vi "Format Serial Data.vi"(0 "Time Stamp":timestamp, 5 "Bus Time":timestamp, 7 "Rail":i32, 9 "String":string, 11 "Error IN":errorcluster, 12 "#of Element Read":i32) -> (4 "Formatted Data":string[](array[string]), 15 "Error OUT":errorcluster)   [LabVIEW 2011]
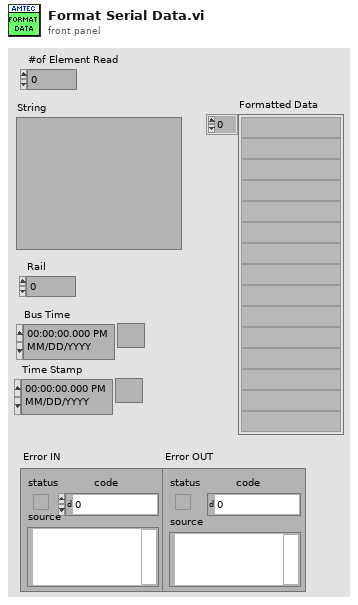
[diagram p1: front panel]
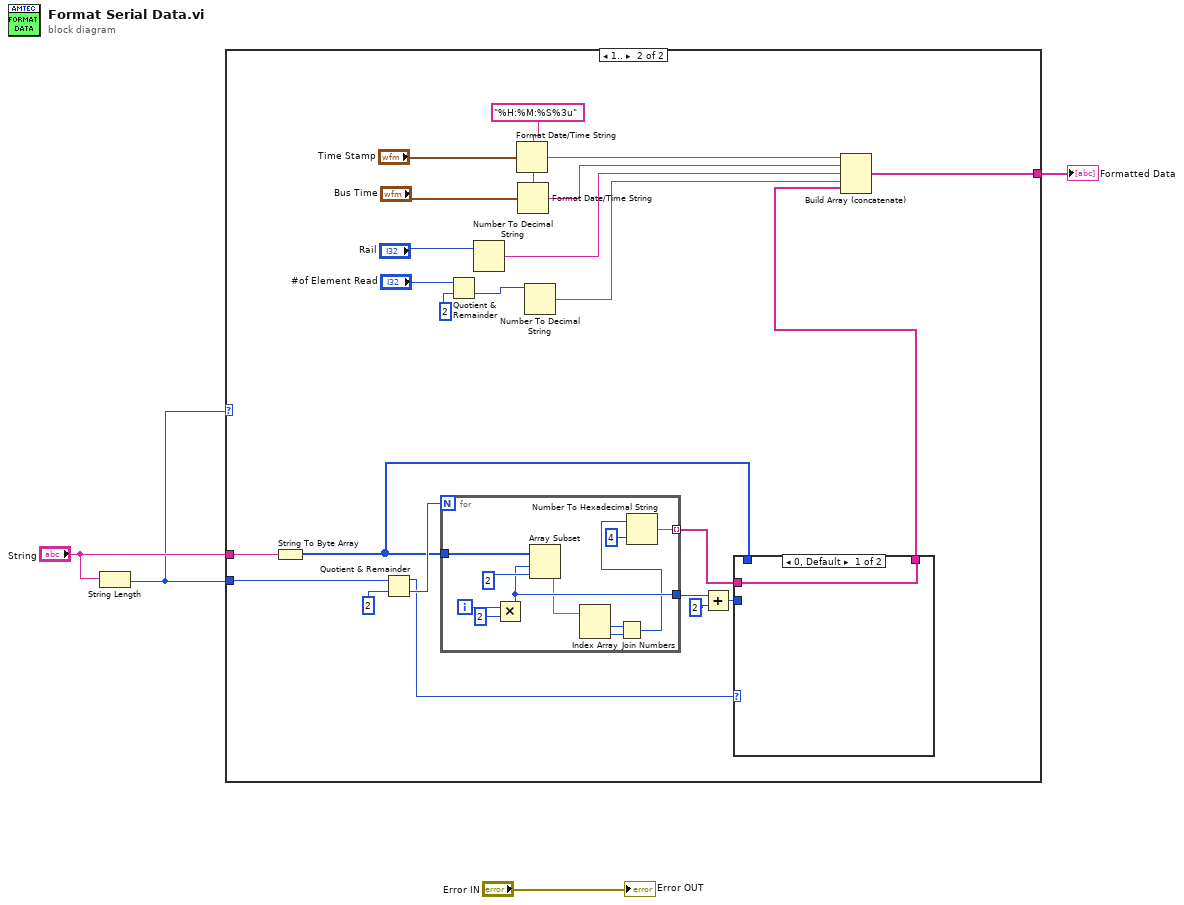
[diagram p0: block diagram]
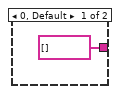
[diagram p2: hidden frame]
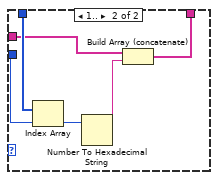
[diagram p3: hidden frame]
diagram:
  n1 = String Length(string="String") -> (length=w1:i32)
  n2 = case shown="1.." w1 {
    tunnel: w1 -> [_ w20]
    tunnel: "String" -> [_ w17]
    tunnel: [string[] [] w9] -> w2
    frame 0, Default {
    }
    frame 1.. {
      w25 = "%H:%M:%S%3u" ("time format string (%c)")
      n3 = String To Byte Array(string=w17) -> (unsigned byte array=w14:u8[])
      n4 = Quotient & Remainder(x=w20, y=2) -> (x-y*floor(x/y)=w12:i32, floor(x/y)=w18:i32)
      n5 = for {
        N: w18 -> [_]
        tunnel: w14 -> [w46]
        tunnel: [w42] -> w16
        tunnel: [w41] -> w11 mode=indexing
        i -> [w45]
        n6 = Multiply(x=w45, y=2) -> (x*y=w42:i32)
        n7 = Array Subset(array=w46, index=w42, length=2 ("y")) -> (w39:u8[])
        n8 = Index Array(array=w39) -> (element #1=w38:u8, element #2=w37:u8)  [unwired: 2 in]
        n9 = Join Numbers(hi=w38, lo=w37) -> ((hi.lo)=w36:u16)
        n10 = Number To Hexadecimal String(1:i16 4 ("width (-)"), 2:w36) -> (0:w41:string)
      }
      n11 = Quotient & Remainder(x="#of Element Read", y=2) -> (floor(x/y)=w6:i32)  [unwired: 1 out]
      n12 = Number To Decimal String(number="Rail") -> (decimal integer string=w22:string)  [unwired: 1 in]
      n13 = Format Date/Time String(time format string (%c)=w25, seconds (now)="Time Stamp") -> (date/time string=w27:string)  [unwired: 1 in]
      n14 = Format Date/Time String(time format string (%c)=w25, seconds (now)="Bus Time") -> (date/time string=w24:string)  [unwired: 1 in]
      n15 = Number To Decimal String(number=w6) -> (decimal integer string=w21:string)  [unwired: 1 in]
      n16 = Add(x=w16, y=2) -> (x+y=w13:i32)
      n17 = case shown="0, Default" w12 {
        tunnel: w14 -> [_ w35]
        tunnel: w13 -> [_ w34]
        tunnel: w11 -> [w29 w32]
        tunnel: [w29 w30] -> w10
        frame 0, Default {
        }
        frame 1.. {
          n18 = Index Array(array=w35, index=w34) -> (element=w33:u8)
          n19 = Number To Hexadecimal String(2:w33) -> (0:w31:string)  [unwired: 1 in]
          n20 = Build Array (concatenate)(w32, w31) -> (w30:string[])
        }
      }
      n21 = Build Array (concatenate)(w27, w24, w22, w21, w10) -> (w9:string[])
    }
  }
  "Formatted Data" <- w2
  "Error OUT" <- "Error IN"
